vi "FB_MFA_Read_Z_Latch1 - NxtMv.vi"() -> (3 "EncoderZLatch":bool)   [LabVIEW 2018]
panel:
  out "AAABuild":i32
  out "error AAABuild":errorcluster
  out "error SetUSBlink":errorcluster
  out "AAABuild 2":i32
  in  "error in":errorcluster
  in  "MintController 2":refnum<k7>(container)
  out "error Z Latch":errorcluster
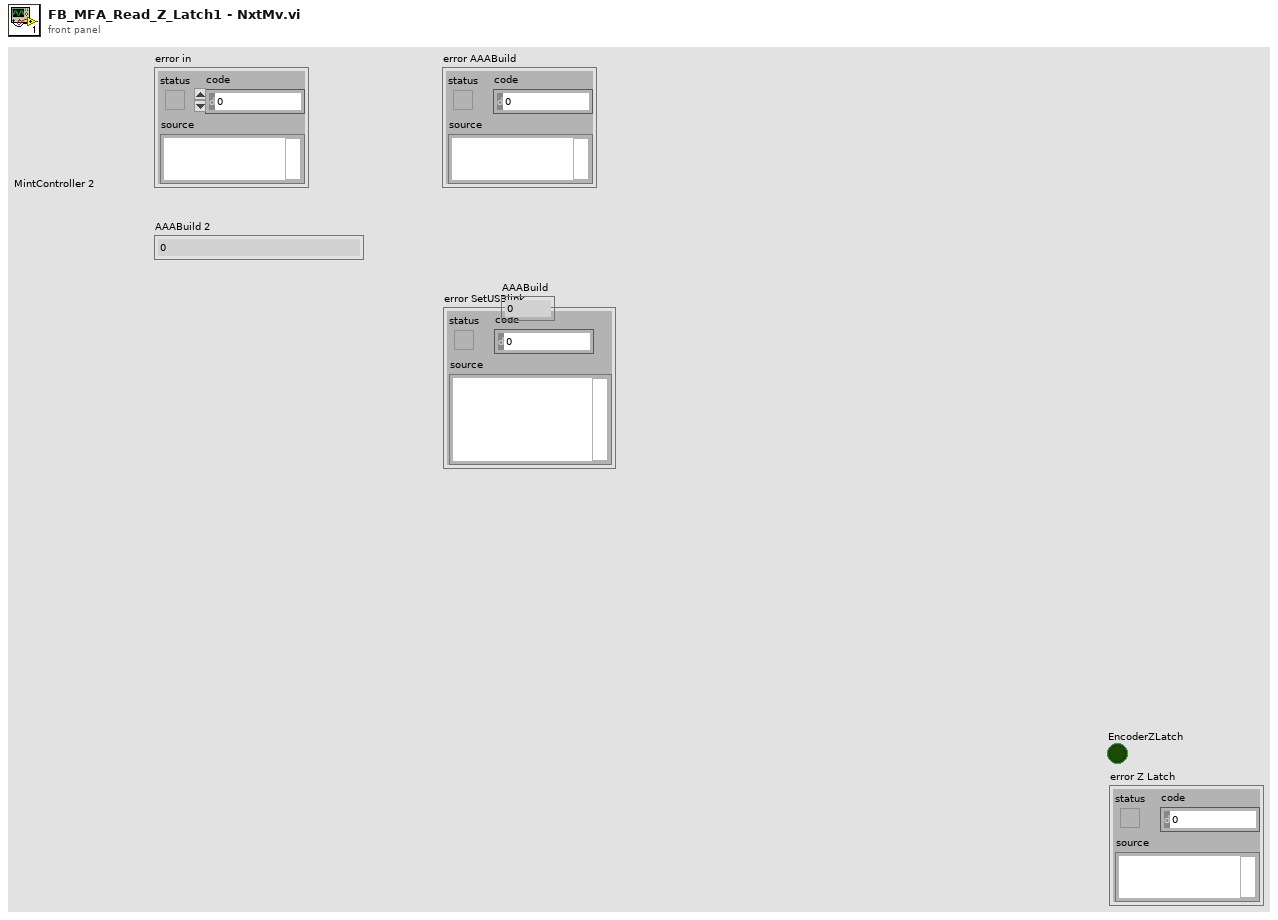
[diagram p1: front panel]
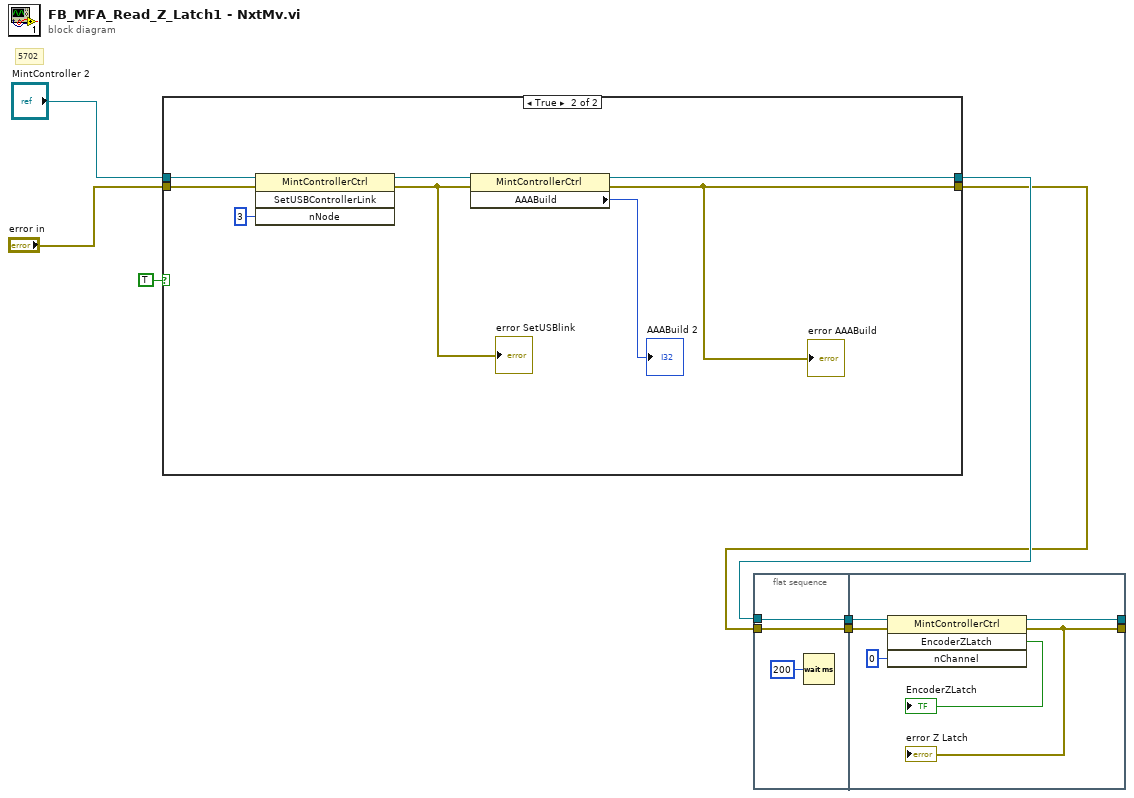
[diagram p0: block diagram]
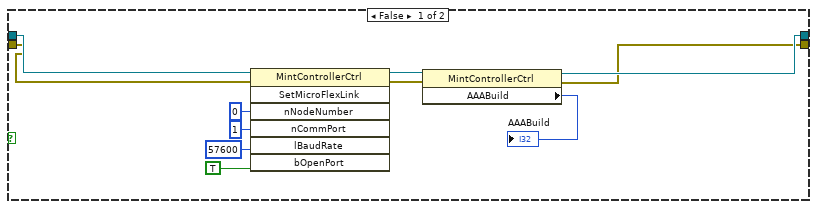
[diagram p2: hidden frame]
diagram:
  # "5702"
  n1 = case shown="True" TRUE {
    tunnel: "MintController 2" -> [w11 w26]
    tunnel: "error in" -> [w10 w25]
    tunnel: [w9 w20] -> w3
    tunnel: [w8 w19] -> w2
    frame False {
      n2 = invoke class="MintControllerCtrl" method="SetMicroFlexLink"(reference=w11, error in=w10, "nNodeNumber"=i16 0, "nCommPort"=i16 1, "lBaudRate"=57600, "bOpenPort"=TRUE) -> (reference out=w18:refnum<k7>, error out=w13:errorcluster)  [unwired: 1 in, 5 out]
      n3 = property class="MintControllerCtrl"(reference=w18, error in=w13) -> (reference out=w9:refnum<k7>, error out=w8:errorcluster, "AAABuild"=→"AAABuild":i32)
    }
    frame True {
      n4 = invoke class="MintControllerCtrl" method="SetUSBControllerLink"(reference=w26, error in=w25, "nNode"=i16 3) -> (reference out=w22:refnum<k7>, error out=w21:errorcluster)  [unwired: 1 in, 2 out]
      "error SetUSBlink" <- w21
      n5 = property class="MintControllerCtrl"(reference=w22, error in=w21) -> (reference out=w20:refnum<k7>, error out=w19:errorcluster, "AAABuild"=→"AAABuild 2":i32)
      "error AAABuild" <- w19
    }
  }
  n6 = flat-sequence {
    tunnel: w3 -> [w28]
    tunnel: [w28] -> w7
    tunnel: w2 -> [w27]
    tunnel: [w27] -> w6
    tunnel: [w34] -> _
    tunnel: [w33] -> _
    tunnel: w7 -> [w32]
    tunnel: w6 -> [w31]
    frame #0 {
      n7 = Wait (ms)(milliseconds to wait=u32 200) -> ()  [unwired: 1 out]
    }
    frame #1 {
      n8 = invoke class="MintControllerCtrl" method="EncoderZLatch"(reference=w32, error in=w31, "nChannel"=i16 0 ("nBank")) -> (reference out=w34:refnum<k7>, error out=w33:errorcluster, "EncoderZLatch"=→"EncoderZLatch":bool)  [unwired: 1 in, 1 out]
      "error Z Latch" <- w33
    }
  }
